vi "Init Actor.vi"() -> (3 "Actor":refnum<class "Actor.lvclass">)   [LabVIEW 2020, in "_Template.lvlib" / "Templates.lvlib" / "{{Name}}Actor.lvlib"]
uses:
  {{Name}}Actor.lvlib
  {{Name}}Actor/{{Name}}Actor.lvclass
  jettl/jettl/Actor/Actor.lvclass
panel:
  # "This front panel should not be manipulated."
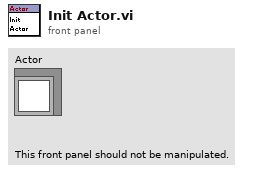
[diagram p1: front panel]
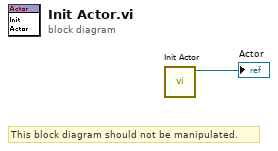
[diagram p0: block diagram]
diagram:
  # "This block diagram should not be manipulated."
  n1 = call "Init Actor.vi"() -> ("TEMPLATE Actor out"=→"Actor":refnum<class "{{Name}}Actor.lvclass">)  [unwired: 11 in]
